vi "User Event Ref FGV.vi"(7 "Command":T1=enum."Get Event Ref", 8 "error in (no error)":errorcluster) -> (0 "error out":errorcluster, 3 "User Event":refnum<user-event>)   [LabVIEW 2010, in "Template Module.lvlib"]
uses:
  Template Module.lvlib
  User Event Message Enum.ctl
  User Event Message Cluster.ctl
  Event Ref FGV Command Enum.ctl
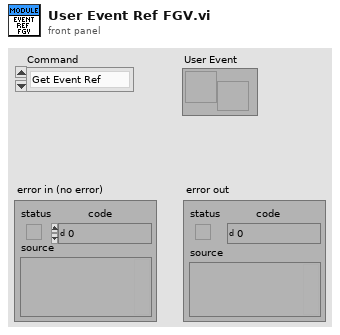
[diagram p1: front panel]
types:
  T1 = typedef "Template Module.lvlib/Event Ref FGV Command Enum.ctl" = enum16{"Create Event", "Get Event Ref", "Release Event"}
  T2 = typedef "Template Module.lvlib/User Event Message Cluster.ctl" = cluster{"Enum":T3, "Data":variant}
  T3 = typedef "Template Module.lvlib/User Event Message Enum.ctl" = enum16{"Event 1"}
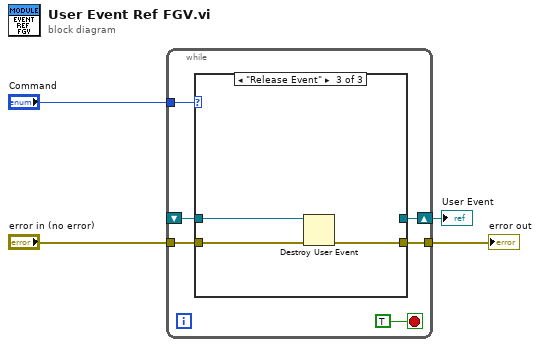
[diagram p0: block diagram]
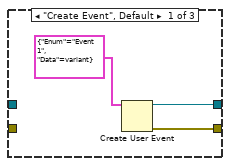
[diagram p2: hidden frame]
diagram:
  n1 = while {
    tunnel: "Command" -> [w9]
    shift-right: [w8] -> w1
    shift-left: _ -> [w7]
    tunnel: [w6] -> w3
    tunnel: "error in (no error)" -> [w5]
    stop <- TRUE stop-if-true
    n2 = case shown="\"Release Event\"" w9 {
      tunnel: [w13 w15 _] -> w8
      tunnel: w7 -> [_ w15 w18]
      tunnel: [w12 w14 w16] -> w6
      tunnel: w5 -> [_ w14 w17]
      frame "Create Event", Default {
        n3 = Create User Event(user event datatype=T2 {"Enum"=enum."Event 1", "Data"=variant} ("Cluster")) -> (user event=w13:refnum<user-event>, error out=w12:errorcluster)  [unwired: 1 in]
      }
      frame "Get Event Ref" {
      }
      frame "Release Event" {
        n4 = Destroy User Event(user event=w18, error in=w17) -> (error out=w16:errorcluster)
      }
    }
  }
  "error out" <- w3
  "User Event" <- w1
